vi "Autonomous.vi"() -> ()   [LabVIEW 2014]
panel:
  in  "script":dbl[][](array[numeric])
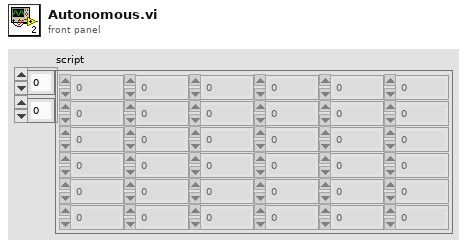
[diagram p1: front panel]
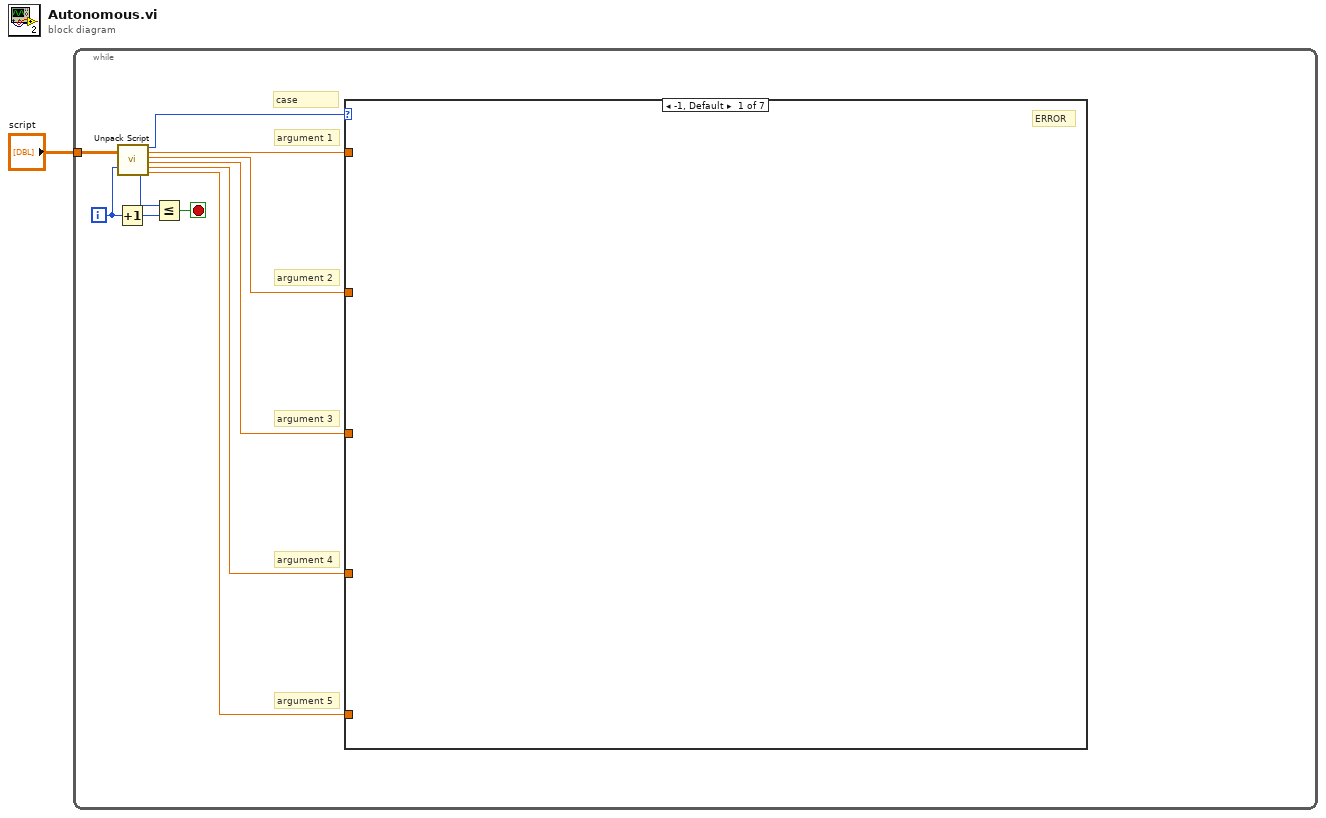
[diagram p0: block diagram]
diagram:
  n1 = while {
    tunnel: "script" -> [w12]
    i -> [w11]
    stop <- w8 stop-if-true
    # "case"
    # "argument 5"
    # "argument 4"
    # "argument 3"
    # "argument 2"
    # "argument 1"
    n2 = Increment(x=w11) -> (x+1=w10:i32)
    n3 = call "Unpack Script.vi"("script"=w12, "index"=w11) -> ("# of primitives"=w9:i32, "primitive"=w7:i32, "argument 1"=w6:dbl, "argument 2"=w5:dbl, "argument 3"=w4:dbl, "argument 4"=w3:dbl, "argument 5"=w2:dbl)  [unwired: 11 in]
    n4 = Less Or Equal?(x=w9, y=w10) -> (x <= y?=w8:bool)
    n5 = case shown="-1, Default" w7 {
      tunnel: w6 -> [_ _ _ _ _ _ _]
      tunnel: w5 -> [_ _ _ _ _ _ _]
      tunnel: w4 -> [_ _ _ _ _ _ _]
      tunnel: w3 -> [_ _ _ _ _ _ _]
      tunnel: w2 -> [_ _ _ _ _ _ _]
      frame -1, Default {
        # "ERROR"
      }
      frame 0 {
        # "delay (seconds)"
        # "DELAY"
      }
      frame 1 {
        # "distance (in.)"
        # "direction (0-360)"
        # "speed (-1 to 1)"
        # "DRIVE"
      }
      frame 3 {
        # "distance (in.)"
        # "speed (0-1)"
        # "INTAKE"
      }
      frame 4 {
        # "speed (0-1)"
        # "level"
        # "LIFT"
      }
      frame 5 {
        # "distance (in.)"
        # "speed (0-1)"
        # "EJECT"
      }
      frame 6 {
        # "speed (0-1)"
        # "level"
        # "distance (in.)"
        # "direction (0-360)"
        # "speed (-1 to 1)"
        # "DRIVE AND LIFT"
      }
    }
  }
